vi "NanotecSMCPDDriver.get positioning mode.vi"(0 "VISA resource name":refnum<visa-resource-name>, 1 "contollerID":i32=-1, 5 "error in (no error)":errorcluster) -> (14 "VISA resource name out":refnum<visa-resource-name>, 15 "contollerID out":i32=-1, 17 "positioningMode":T1, 19 "error out":errorcluster)   [LabVIEW 2014, in "NanotecSMCPDDriver.lvlib"]
doc: "Gets the positioning mode of the motor (relative, absolute, ...)"
uses:
  NanotecSMCPDDriver.lvlib
  NanotecSMCPDDriver.positioning mode types.ctl
  NanotecSMCPDDriver.controller mode types.ctl
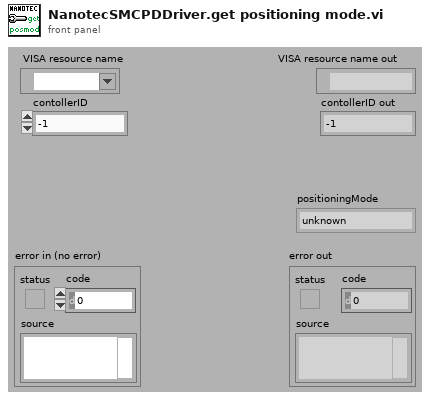
[diagram p1: front panel]
types:
  T1 = typedef "NanotecSMCPDDriver.lvlib/NanotecSMCPDDriver.positioning mode types.ctl" = enum16{"unknown", "relative positioning", "absolute positioning", "internal referencing", "external referencing"}
  T2 = typedef "NanotecSMCPDDriver.lvlib/NanotecSMCPDDriver.controller mode types.ctl" = enum16{"unknown", "position", "speed", "flagPosition", "clockDirection", "analog", "joystick"}
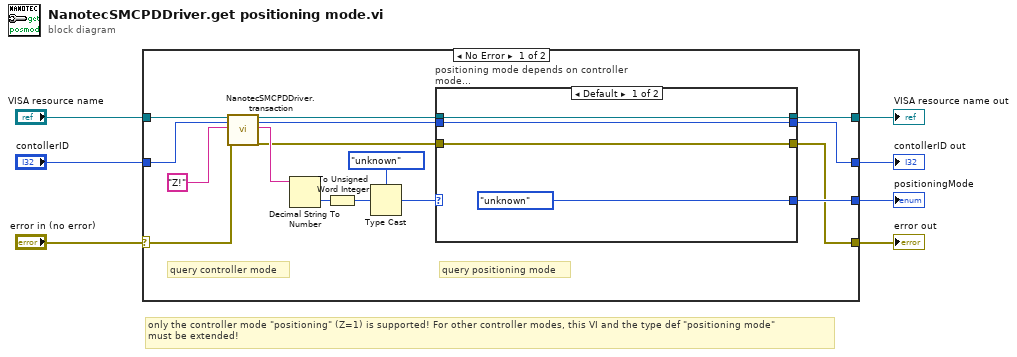
[diagram p0: block diagram]
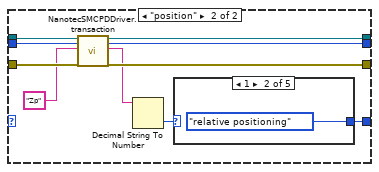
[diagram p2: hidden frame]
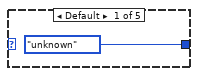
[diagram p3: hidden frame]
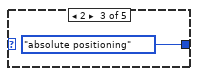
[diagram p4: hidden frame]
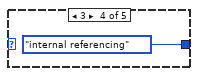
[diagram p5: hidden frame]
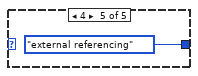
[diagram p6: hidden frame]
diagram:
  # "only the controller mode \"positioning\" (Z=1) is supported! For other controller modes, this VI and the type def \"positioning mode\"\nmust be extended!"
  n1 = case shown="No Error" "error in (no error)" {
    selector: "error in (no error)" -> [w19 w43]
    tunnel: [w12 w45] -> w7
    tunnel: [w9 w43] -> w6
    tunnel: "VISA resource name" -> [w23 w45]
    tunnel: "contollerID" -> [w21 w44]
    tunnel: [w11 w44] -> w3
    tunnel: [w10 _] -> w2
    frame No Error {
      # "query positioning mode"
      # "query controller mode"
      n2 = call "NanotecSMCPDDriver.transaction.vi"("VISAresource"=w23, "contollerID"=w21, "commandString"="Z!", "error in (no error)"=w19) -> ("VISAresource out"=w14:refnum<visa-resource-name>, "contollerID out"=w13:i32, "response"=w20:string, "error out"=w15:errorcluster)  [unwired: 10 in, 2 out]
      n3 = Decimal String To Number(string=w20) -> (number=w18:i32)  [unwired: 2 in, 1 out]
      n4 = To Unsigned Word Integer(number=w18) -> (unsigned 16bit integer=w8:u16)
      n5 = Type Cast(type=NanotecSMCPDDriver.controller_mode_types."unknown" ("controllerMode"), x=w8) -> (*(type *) &x=w16:T2)
      n6 = case "positioning mode depends on controller mode..." shown="Default" w16 {
        tunnel: w15 -> [w24 w33]
        tunnel: w14 -> [w27 w37]
        tunnel: w13 -> [w26 w36]
        tunnel: [w27 w35] -> w12
        tunnel: [w26 w34] -> w11
        tunnel: [NanotecSMCPDDriver.positioning_mode_types."unknown" ("positioningMode type") w28] -> w10
        tunnel: [w24 w32] -> w9
        frame Default {
        }
        frame "position" {
          n7 = call "NanotecSMCPDDriver.transaction.vi"("VISAresource"=w37, "contollerID"=w36, "commandString"="Zp", "error in (no error)"=w33) -> ("VISAresource out"=w35:refnum<visa-resource-name>, "contollerID out"=w34:i32, "response"=w30:string, "error out"=w32:errorcluster)  [unwired: 10 in, 2 out]
          n8 = Decimal String To Number(string=w30) -> (number=w29:i32)  [unwired: 2 in, 1 out]
          n9 = case shown="1" w29 {
            tunnel: [NanotecSMCPDDriver.positioning_mode_types."unknown" ("positioningMode type") NanotecSMCPDDriver.positioning_mode_types."relative positioning" ("positioningMode type") NanotecSMCPDDriver.positioning_mode_types."absolute positioning" ("positioningMode type") NanotecSMCPDDriver.positioning_mode_types."internal referencing" ("positioningMode type") NanotecSMCPDDriver.positioning_mode_types."external referencing" ("positioningMode type")] -> w28
            frame Default {
            }
            frame 1 {
            }
            frame 2 {
            }
            frame 3 {
            }
            frame 4 {
            }
          }
        }
      }
    }
    frame Error {
    }
  }
  "positioningMode" <- w2
  "VISA resource name out" <- w7
  "error out" <- w6
  "contollerID out" <- w3
